vi "OE2012&OE2022_Query Data.vi"(0 "VISA resource name":refnum<visa-resource-name>, 5 "Connection ID in":refnum<k5>, 7 "Remote Mode":u16(ring) items=["USB", "RS232", "GPIB", "Ethernet"], 11 "Error in (no error)":errorcluster caption="error out（no error）") -> (4 "VISA resource  out":refnum<visa-resource-name>, 6 "Connection ID out":refnum<k5>, 8 "Parameter Values":T1, 10 "Output String":string, 15 "Error out":errorcluster caption="error out")   [LabVIEW 2011]
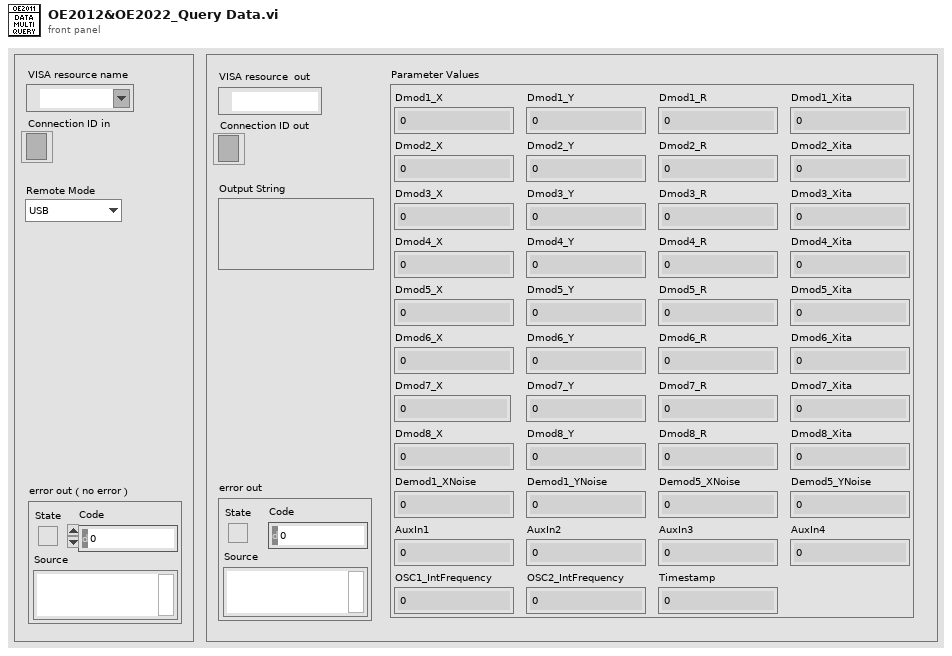
[diagram p1: front panel]
types:
  T1 = cluster{"Dmod1_X":dbl, "Dmod1_Y":dbl, "Dmod1_R":dbl, "Dmod1_Xita":dbl, "Dmod2_X":dbl, "Dmod2_Y":dbl, "Dmod2_R":dbl, "Dmod2_Xita":dbl, "Dmod3_X":dbl, "Dmod3_Y":dbl, "Dmod3_R":dbl, "Dmod3_Xita":dbl, "Dmod4_X":dbl, "Dmod4_Y":dbl, "Dmod4_R":dbl, "Dmod4_Xita":dbl, "Dmod5_X":dbl, "Dmod5_Y":dbl, "Dmod5_R":dbl, "Dmod5_Xita":dbl, "Dmod6_X":dbl, "Dmod6_Y":dbl, "Dmod6_R":dbl, "Dmod6_Xita":dbl, "Dmod7_X":dbl, "Dmod7_Y":dbl, "Dmod7_R":dbl, "Dmod7_Xita":dbl, "Dmod8_X":dbl, "Dmod8_Y":dbl, "Dmod8_R":dbl, "Dmod8_Xita":dbl, "Demod1_XNoise":dbl, "Demod1_YNoise":dbl, "Demod5_XNoise":dbl, "Demod5_YNoise":dbl, "OSC1_IntFrequency":dbl, "OSC2_IntFrequency":dbl, "AuxIn1":dbl, "AuxIn2":dbl, "AuxIn3":dbl, "AuxIn4":dbl, "Timestamp":dbl}
  T2 = cluster{dbl, dbl, dbl, dbl, dbl, dbl, dbl, dbl, dbl, dbl, dbl, dbl, dbl, dbl, dbl, dbl, dbl, dbl, dbl, dbl, dbl, dbl, dbl, dbl, dbl, dbl, dbl, dbl, dbl, dbl, dbl, dbl, dbl, dbl, dbl, dbl, dbl, dbl, dbl, dbl, dbl, dbl, dbl}
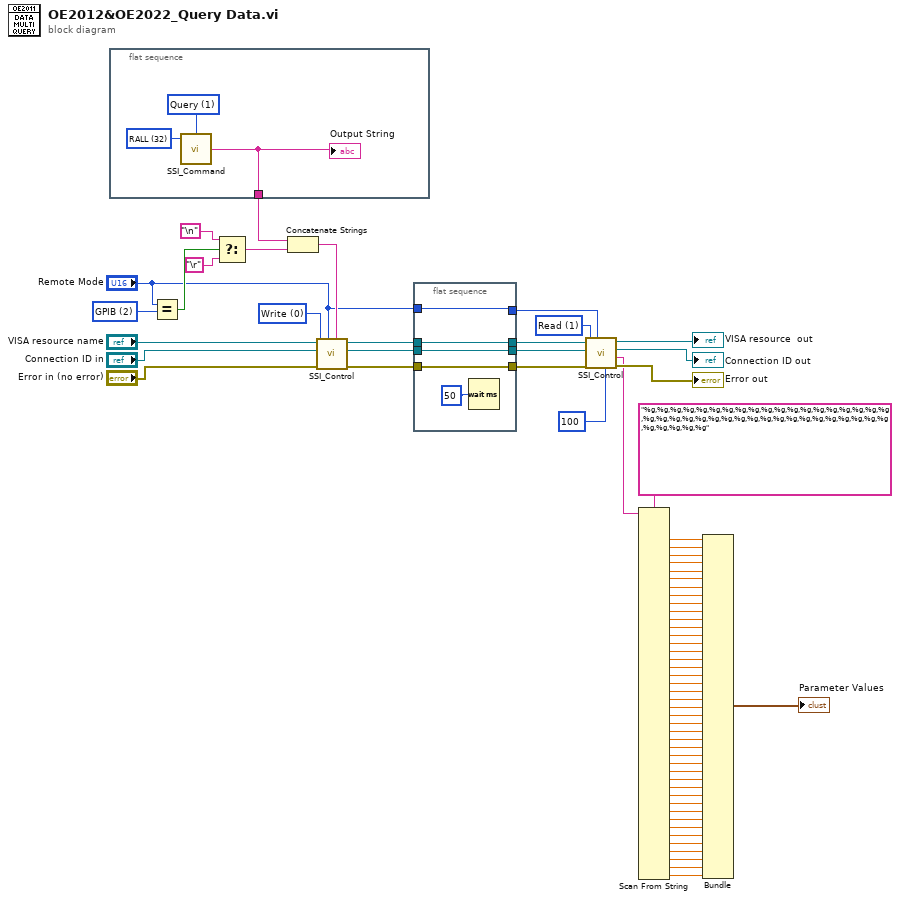
[diagram p0: block diagram]
diagram:
  w60 = u16 2 items=["USB", "RS232", "GPIB", "Ethernet"] ("Remote Mode")
  w65 = u16 1 items=["Write", "Read"] ("Control")
  w70 = u16 0 items=["Write", "Read"] ("Control")
  n1 = flat-sequence {
    tunnel: [w71] -> w50
    frame #0 {
      w73 = u16 32 items=["ISRC", "IGND", "ICPL", "ILIN", "PHAS", "FMOD", "RSLP", "FREQ", "SWPT", "SLLM", "SULM", "SSLL", "SSLG", "STLM", "SWRM", "IRNG", "SENS", "RMOD", "OFLT", "OFSL", "SYNC", "DMOD", "HARM", "DARB", "SWVT", "SLVL", "SVLL", "SVUL", "SVSL", "SVSG", "SVTM", "SVRM", "RALL", "SNAP", "OUTP", "OAUX", "COUT", "CAUX", "COFP", "CEXP", "FPOP", "OEXP", "*IDN", "*RST", "OVLD", "INOV", "GNOV", "*PLL", "SSET", "RSET", "AGAN", "APHS", "ARSV", "ASCL", "EQCD", "EQCS", "SPED", "SRAT", "SLEN", "SSLE", "STRG", "SPRM", "STRD", "PAUS", "RSET", "SPTS", "TRCA", "TEMP", "RSTU", "INHZ", "DEQU", "SADD", "ARNG", "CSPE", "ISRCD", "IGNDD", "ICPLD", "ILIND", "PHASD", "FMODD", "RSLPD", "FREQD", "SWPTD", "SLLMD", "SULMD", "SSLLD", "SSLGD", "STLMD", "SWRMD", "SENSD", "RMODD", "OFLTD", "OFSLD", "SYNCD", "HARMD", "EQCDD", "EQCSD", "SNAPD", "OUTPD", "SWVTD", "SLVLD", "SVLLD", "SVULD", "SVSLD", "SVSGD", "SVTMD", "SVRMD", "SVDCD", "ARSVD", "AGAND", "APHSD", "ASCLD", "FPOPD", "CAUXD", "OEXPD", "SPEDD", "SRATD", "SLEND", "SSLED", "STRGD", "SPRMD", "STRDD", "PAUSD", "RESTD", "SPTSD", "TRCAD", "*IDND", "*RSTD", "INOVD", "GNOVD", "*PLLD", "SSETD", "RSETD", "RALLD"] ("Command Type")
      w72 = u16 1 items=["Set", "Query"] ("Opera")
      n2 = call "SSI_Command.vi"("Opera"=w72, "Command Type"=w73) -> ("Output string"=w71:string)  [unwired: 2 in]
      "Output String" <- w71
    }
  }
  n3 = Equal?(x="Remote Mode", y=w60) -> (x = y?=w55:bool)
  n4 = Select(t="\n", s=w55, f="\r") -> (s? t:f=w58:string)
  n5 = Concatenate Strings(w50, w58) -> (w56:string)
  n6 = call "SSI_Control.vi"("Write Buffer"=w56, "Remote Mode"="Remote Mode", "Error in (no error)"="Error in (no error)", "Control"=w70, "Connection ID in"="Connection ID in", "VISA resource name"="VISA resource name") -> ("Error out"=w68:errorcluster, "Connection ID out"=w49:refnum<k5>, "VISA resource  out"=w69:refnum<visa-resource-name>)  [unwired: 2 in, 1 out]
  n7 = flat-sequence {
    tunnel: w69 -> [w78]
    tunnel: w68 -> [w77]
    tunnel: [w78] -> w67
    tunnel: [w77] -> w66
    tunnel: [w75] -> w64
    tunnel: "Remote Mode" -> [w75]
    tunnel: w49 -> [w74]
    tunnel: [w74] -> w48
    frame #0 {
      n8 = Wait (ms)(milliseconds to wait=u32 50 ("等待时间（毫秒）")) -> ()  [unwired: 1 out]
    }
  }
  n9 = call "SSI_Control.vi"("Tineout"=100, "Remote Mode"=w64, "Error in (no error)"=w66, "Control"=w65, "Connection ID in"=w48, "VISA resource name"=w67) -> ("Error out"=→"Error out":errorcluster, "Read Buffer"=w3:string, "Connection ID out"=→"Connection ID out":refnum<k5>, "VISA resource  out"=→"VISA resource  out":refnum<visa-resource-name>)  [unwired: 2 in]
  n10 = Scan From String(format string="%g,%g,%g,%g,%g,%g,%g,%g,%g,%g,%g,%g,%g,%g,%g,%g,%g,%g,%g,%g,%g,%g,%g,%g,%g,%g,%g,%g,%g,%g,%g,%g,%g,%g,%g,%g,%g,%g,%g,%g,%g,%g,%g" ("格式字符串"), input string=w3) -> (output 1=w47:dbl, output 2=w46:dbl, output 3=w45:dbl, output 4=w44:dbl, output 5=w43:dbl, output 6=w42:dbl, output 7=w41:dbl, output 8=w40:dbl, output 9=w39:dbl, output 10=w38:dbl, output 11=w37:dbl, output 12=w36:dbl, output 13=w35:dbl, output 14=w34:dbl, output 15=w6:dbl, output 16=w7:dbl, output 17=w5:dbl, output 18=w8:dbl, output 19=w9:dbl, output 20=w10:dbl, output 21=w11:dbl, output 22=w12:dbl, output 23=w13:dbl, output 24=w14:dbl, output 25=w15:dbl, output 26=w16:dbl, output 27=w17:dbl, output 28=w18:dbl, output 29=w19:dbl, output 30=w20:dbl, output 31=w21:dbl, output 32=w22:dbl, output 33=w23:dbl, output 34=w24:dbl, output 35=w25:dbl, output 36=w26:dbl, output 37=w27:dbl, output 38=w28:dbl, output 39=w29:dbl, output 40=w30:dbl, output 41=w31:dbl, output 42=w32:dbl, output 43=w33:dbl)  [unwired: 45 in, 3 out]
  n11 = Bundle(w47, w46, w45, w44, w43, w42, w41, w40, w39, w38, w37, w36, w35, w34, w6, w7, w5, w8, w9, w10, w11, w12, w13, w14, w15, w16, w17, w18, w19, w20, w21, w22, w23, w24, w25, w26, w27, w28, w29, w30, w31, w32, w33) -> (→"Parameter Values":T2)  [unwired: 1 in]
